vi "JumpBreak.vi"(3 "error in":errorcluster, 4 "Running":bool, 5 "Input Value":dbl, 9 "JumpValue":dbl, 11 "JumpTime":dbl, 12 "JumpAt":dbl) -> (8 "OutputValue":dbl, 14 "error out":errorcluster)   [LabVIEW 2016]
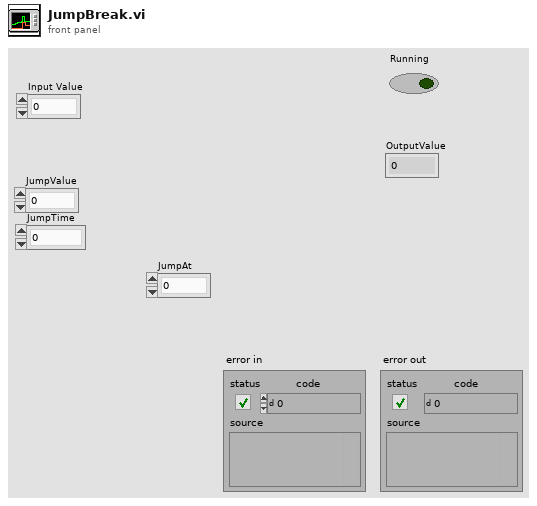
[diagram p1: front panel]
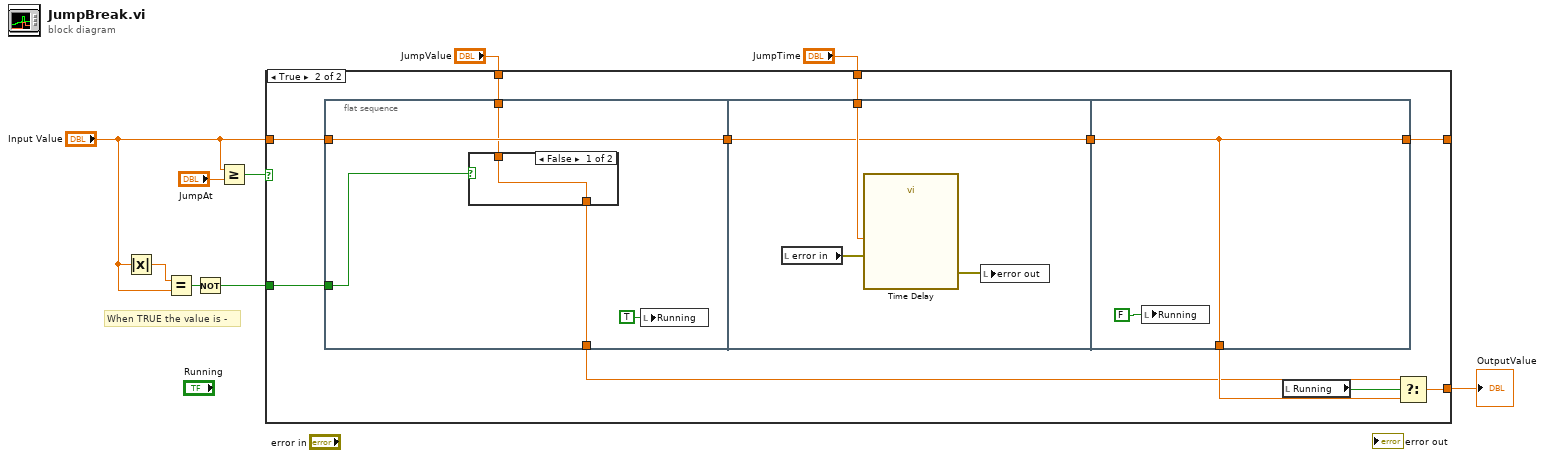
[diagram p0: block diagram]
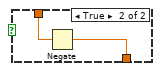
[diagram p3: hidden frame]
diagram:
  # "When TRUE the value is -"
  n1 = Absolute Value(x="Input Value") -> (abs(x)=w5:dbl)
  n2 = Equal?(x=w5, y="Input Value") -> (x = y?=w3:bool)
  n3 = Not(x=w3) -> (.not. x?=w2:bool)
  n4 = Greater Or Equal?(x="Input Value", y="JumpAt") -> (x >= y?=w8:bool)
  n5 = case shown="True" w8 {
    tunnel: [w10 w16] -> _
    tunnel: "Input Value" -> [w10 w17]
    tunnel: "JumpTime" -> [_ w21]
    tunnel: "JumpValue" -> [_ w20]
    tunnel: w2 -> [_ w15]
    tunnel: [w10 w14] -> w1
    frame False {
    }
    frame True {
      n6 = flat-sequence {
        tunnel: w20 -> [w24]
        tunnel: [w26] -> w18
        tunnel: w17 -> [w26]
        tunnel: w15 -> [w25]
        tunnel: [w23] -> w12
        tunnel: w21 -> [w33]
        tunnel: [w32] -> w19
        tunnel: w18 -> [w32]
        tunnel: w19 -> [w35]
        tunnel: [w35] -> w16
        tunnel: [w35] -> w13
        frame #0 {
          n7 = case shown="False" w25 {
            tunnel: w24 -> [w27 w29]
            tunnel: [w27 w28] -> w23
            frame False {
            }
            frame True {
              n8 = Negate(x=w29) -> (-x=w28:dbl)
            }
          }
          n9 = local write "Running"(TRUE) -> ()
        }
        frame #1 {
          n10 = local read "error in"() -> (w30:errorcluster)
          n11 = call "Time Delay"("error in (no error)"=w30, "Delay Time (s)"=w33) -> ("error out"=w31:errorcluster)  [unwired: 9 in]
          n12 = local write "error out"(w31) -> ()
        }
        frame #2 {
          n13 = local write "Running"(FALSE) -> ()
        }
      }
      n14 = local read "Running"() -> (w11:bool)
      n15 = Select(t=w12, s=w11, f=w13) -> (s? t:f=w14:dbl)
    }
  }
  "OutputValue" <- w1
